vi "LVtest.vi"() -> ()   [LabVIEW 2014]
panel:
  in  "stop":bool
  in  "Boolean 2":bool
  out "Boolean":bool
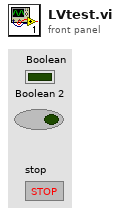
[diagram p1: front panel]
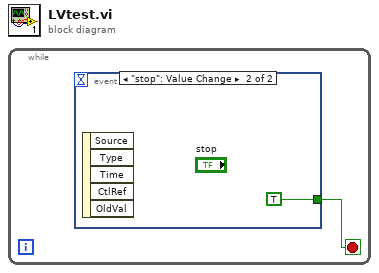
[diagram p0: block diagram]
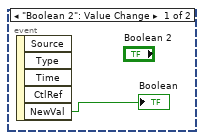
[diagram p2: hidden frame]
diagram:
  n1 = while {
    stop <- w1 stop-if-true
    n2 = event shown="[1] \"stop\": Value Change" {
      selector: _ -> [_ _]
      dyn-events: _ -> [_ _]
      timeout: _ -> [_ _]
      tunnel: [_ TRUE] -> w1
      event "Boolean 2": Value Change {
        n3 = event-data() -> ("NewVal"=→"Boolean":bool)  [unwired: 1 in, 4 out]
      }
      event "stop": Value Change {
        n4 = event-data() -> ()  [unwired: 1 in, 5 out]
      }
    }
  }
